vi "Broadcast Channel Data.vi"(8 "error in (no error)":errorcluster, 11 "Output Channel in":refnum<class "Output Channel.lvclass">) -> (0 "error out":errorcluster, 3 "Output Channel out":refnum<class "Output Channel.lvclass">)   [LabVIEW 2015, in "Output Channel.lvlib" / "Output Channel.lvclass"]
uses:
  Output Channel.lvclass
  <vilib>/ActorFramework/Actor/Actor.lvclass/Actor.ctl
  <vilib>/ActorFramework/Message Enqueuer/Message Enqueuer.lvclass/Message Enqueuer.ctl
  <vilib>/ActorFramework/Message Enqueuer/Init from Existing Queue.vi
  Channel/Channel/Channel.lvclass
  <vilib>/ActorFramework/Message Enqueuer/Message Enqueuer.lvclass
  Channel/ChannelData.lvclass
  <vilib>/ActorFramework/Actor/Actor.lvclass
  Sequencer/Sequencer Messages/Update Channel Data Msg/Update Channel Data Msg.lvclass
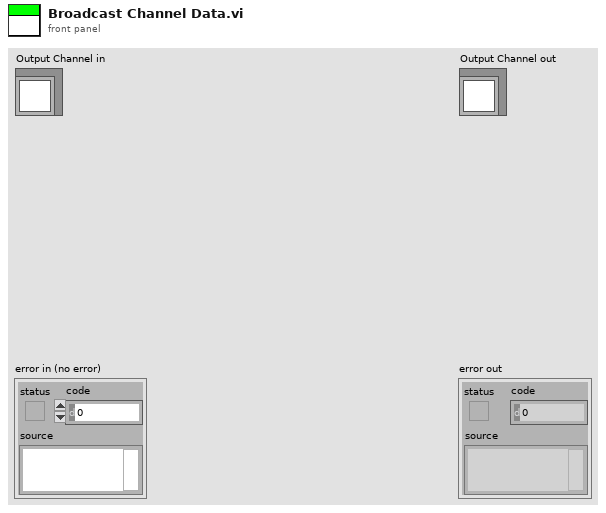
[diagram p1: front panel]
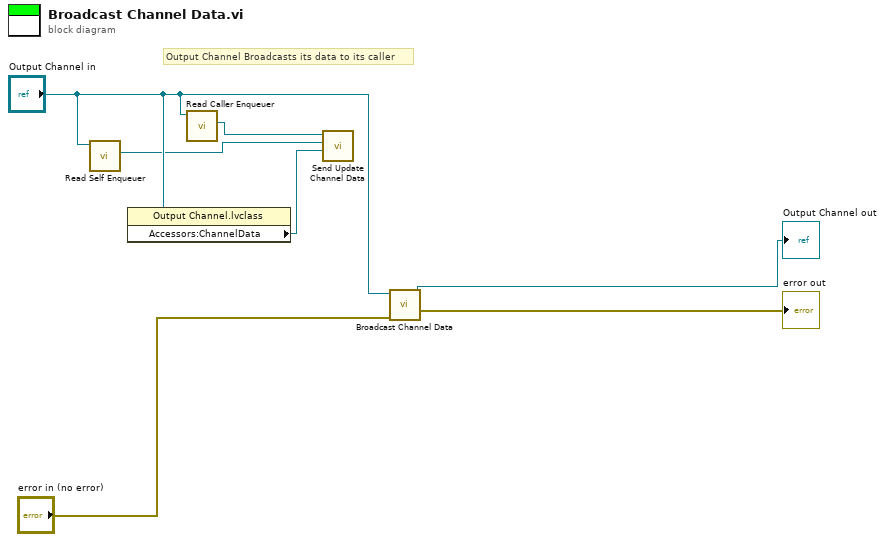
[diagram p0: block diagram]
diagram:
  # "Output Channel Broadcasts its data to its caller"
  n1 = call <vilib>:"Read Self Enqueuer.vi"("Actor"="Output Channel in") -> ("Self Enqueuer"=w1:refnum<class "Message Enqueuer.lvclass">)  [unwired: 10 in]
  n2 = property class="Output Channel.lvclass"(reference="Output Channel in") -> ("Accessors:ChannelData"=w2:refnum<class "ChannelData.lvclass">)  [unwired: 1 in, 2 out]
  n3 = call <vilib>:"Read Caller Enqueuer.vi"("Actor"="Output Channel in") -> ("Caller Enqueuer"=w3:refnum<class "Message Enqueuer.lvclass">)  [unwired: 10 in]
  n4 = call "Send Update Channel Data.vi"("ChannelData"=w2, "Channel Enququer"=w1, "Message Enqueuer in"=w3) -> ()  [unwired: 7 in, 2 out]
  n5 = call-parent "Broadcast Channel Data.vi"("error in (no error)"="error in (no error)", "Channel in"="Output Channel in") -> ("error out"=→"error out":errorcluster, "Channel out"=→"Output Channel out":refnum<class "Output Channel.lvclass">)  [unwired: 8 in]
